vi "EASY-Setup Chart.vi"(8 "error in (no error)":errorcluster, 9 "Series":T1={"ChartType"=0, "Name"="", "Palette"=enum."None", "BorderDashStyle"=enum."NotSet", "YAxisType"=enum."Primary", "XAxisType"=enum."Primary", "BorderColor"=0, "Thickness"=0.0, "Color"=11711154, "Alpha"=76, "Marker"={"MarkerStyle"=enum."None", "Size"=0, "Color"=0, "Step"=0}} {"Alpha" scale=0.0..255.0; "ChartType" items=["Point", "FastPoint", "Bubble", "Line", "Spline", "StepLine", "FastLine", "Bar", "StackedBar", "StackedBar100", "Column", "StackedColumn", "StackedColumn100", "Area", "SplineArea", "StackedArea", "StackedArea100", "Pie", "Doughnut", "Stock", "Candlestick", "Range", "SplineRange", "RangeBar", "RangeColumn", "Radar", "Polar", "ErrorBar", "BoxPlot", "Renko", "ThreeLineBreak", "Kagi", "PointAndFigure", "Funnel", "Pyramid"]}, 10 "Chart Options":T3 {"Legend"."BGKalpha" scale=0.0..255.0; "Title"."TitleFontSize" min=4.0 max=100.0}, 11 ".NET MSChart":refnum<k24>(container)) -> (0 "error out":errorcluster, 2 ".net MSChart Series":refnum<k24>, 3 ".NET MSChart":refnum<k24>)   [LabVIEW 2015, in "Graph Extensions MSChart.lvlib"]
uses:
  Graph Extensions MSChart.lvlib
  System.Windows.Forms.DataVisualization
  Controls/Chart.ctl
  Controls/Title.ctl
  Controls/Legend.ctl
  Controls/Series.ctl
  Controls/Marker.ctl
  Controls/3D.ctl
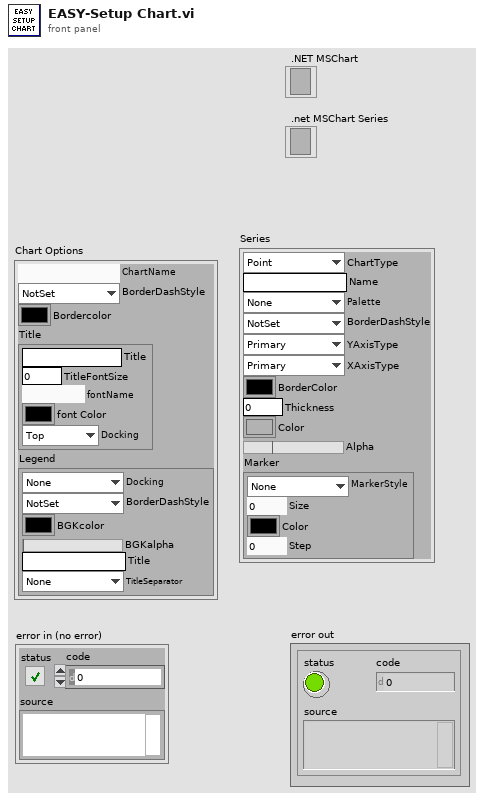
[diagram p1: front panel]
types:
  T1 = typedef "Graph Extensions MSChart.lvlib/Series.ctl" = cluster{"ChartType":i32, "Name":string, "Palette":enum16{"None", "Bright", "Grayscale", "Excel", "Light", "Pastel", "EarthTones", "SemiTransparent", "Berry", "Chocolate", "Fire", "SeaGreen", "BrightPastel"}, "BorderDashStyle":enum16{"NotSet", "Dash", "DashDot", "DashDotDot", "Dot", "Solid"}, "YAxisType":enum16{"Primary", "Secondary"}, "XAxisType":enum16{"Primary", "Secondary"}, "BorderColor":u32, "Thickness":dbl, "Color":u32, "Alpha":u8, "Marker":T2}
  T2 = typedef "Graph Extensions MSChart.lvlib/Marker.ctl" = cluster{"MarkerStyle":enum16{"None", "Square", "Circle", "Diamond", "Triangle", "Cross", "Star4", "Star5", "Star6", "Star10"}, "Size":i32, "Color":u32, "Step":i32}
  T3 = typedef "Graph Extensions MSChart.lvlib/Chart.ctl" = cluster{"ChartName":string, "BorderDashStyle":enum16{"NotSet", "Dash", "DashDot", "DashDotDot", "Dot", "Solid"}, "Bordercolor":u32, "Title":T4, "Legend":T5}
  T4 = typedef "Graph Extensions MSChart.lvlib/Title.ctl" = cluster{"Title":string, "TitleFontSize":dbl, "fontName":string, "font Color":u32, "Docking":enum16{"Top", "Right", "Bottom", "Left"}}
  T5 = typedef "Graph Extensions MSChart.lvlib/Legend.ctl" = cluster{"Docking":enum16{"None", "Top", "Right", "Bottom", "Left"}, "BorderDashStyle":enum16{"NotSet", "Dash", "DashDot", "DashDotDot", "Dot", "Solid"}, "BGKcolor":u32, "BGKalpha":u8, "Title":string, "TitleSeparator":enum16{"None", "Line", "ThickLine", "DoubleLine", "DashLine", "DotLine", "GradientLine", "ThickGradientLine"}}
  T6 = typedef "Graph Extensions MSChart.lvlib/3D.ctl" = cluster{"Enable 3D":bool, "LightStyle":enum16{"None", "Simplistic", "Realistic"}, "PointGapDepth":i32, "PointDepth":i32, "Perspective":i32, "WallWidth":i32}
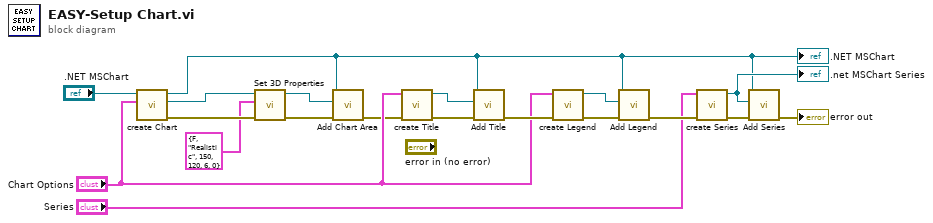
[diagram p0: block diagram]
diagram:
  n1 = call "create Chart.vi"("Chart Options"="Chart Options", ".NET MSChart"=".NET MSChart") -> ("error out"=w5:errorcluster, ".NET MSChart ChartArea"=w6:refnum<k24>, ".NET MSChart"=w2:refnum<k24>)  [unwired: 7 in]
  ".NET MSChart" <- w2
  n2 = call "Set 3D Properties.vi"("error in (no error)"=w5, "3D"=T6 {"Enable 3D"=FALSE, "LightStyle"=enum."Realistic", "PointGapDepth"=150, "PointDepth"=120, "Perspective"=6, "WallWidth"=0}, ".NET MSChart ChartArea"=w6) -> ("error out"=w7:errorcluster, ".NET MSChart ChartArea"=w8:refnum<k24>)  [unwired: 7 in]
  n3 = call "Add Chart Area.vi"("error in (no error)"=w7, ".NET MSChart ChartArea"=w8, ".NET MSChart"=w2) -> ("error out"=w9:errorcluster)  [unwired: 8 in]
  n4 = call "create Title.vi"("error in (no error)"=w9, "Chart Options"="Chart Options") -> ("error out"=w11:errorcluster, ".NET MSChart Title"=w13:refnum<k24>)  [unwired: 8 in]
  n5 = call "Add Title.vi"("error in (no error)"=w11, ".NET MSChart Title"=w13, ".NET MSChart"=w2) -> ("error out"=w12:errorcluster)  [unwired: 8 in]
  n6 = call "create Legend.vi"("error in (no error)"=w12, "Chart Options"="Chart Options") -> ("error out"=w14:errorcluster, ".NET MSChart Legend"=w16:refnum<k24>)  [unwired: 8 in]
  n7 = call "Add Legend.vi"("error in (no error)"=w14, ".NET MSChart Legend"=w16, ".NET MSChart"=w2) -> ("error out"=w15:errorcluster)  [unwired: 8 in]
  n8 = call "create Series.vi"("error in (no error)"=w15, "Series"="Series") -> ("error out"=w17:errorcluster, ".net MSChart Series"=w19:refnum<k24>)  [unwired: 8 in]
  ".net MSChart Series" <- w19
  n9 = call "Add Series.vi"("error in (no error)"=w17, ".net MSChart Series"=w19, ".NET MSChart"=w2) -> ("error out"=→"error out":errorcluster)  [unwired: 8 in]
